vi "Write WebSocket Server Enqueuer.vi"(8 "error in (no error)":errorcluster, 10 "Actor Framework:Message Enqueuer":refnum<class "Message Enqueuer.lvclass">, 11 "WS Test Server in":refnum<class "WS Server Subscriber.lvclass">) -> (0 "error out":errorcluster, 3 "WS Test Server out":refnum<class "WS Server Subscriber.lvclass">)   [LabVIEW 2021, in "Echo Broadcast With Server Manager.lvlib" / "WS Server Subscriber.lvclass"]
uses:
  WS Server Subscriber.lvclass
  <vilib>/ActorFramework/Message Enqueuer/Message Enqueuer.lvclass
  WS Server Subscriber.lvclass/WS Server Subscriber.ctl
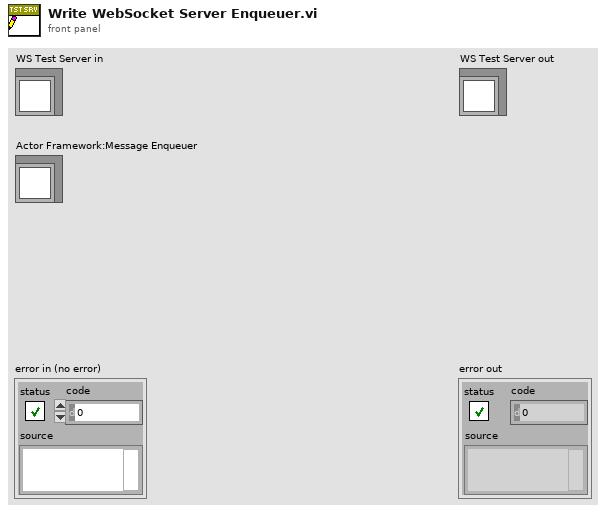
[diagram p1: front panel]
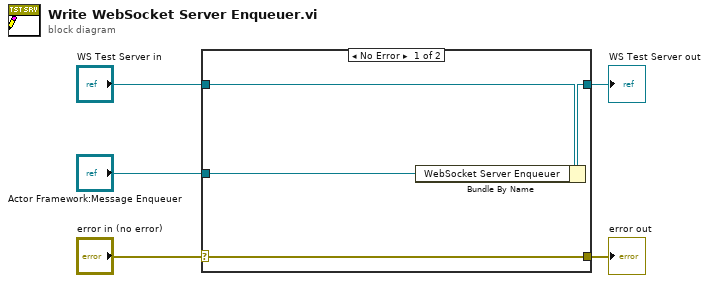
[diagram p0: block diagram]
diagram:
  n1 = case shown="No Error" "error in (no error)" {
    selector: "error in (no error)" -> [w9 w10]
    tunnel: [w9 w10] -> w4
    tunnel: [w7 w11] -> w2
    tunnel: "WS Test Server in" -> [w8 w11]
    tunnel: "Actor Framework:Message Enqueuer" -> [w6 _]
    frame No Error {
      n2 = Bundle By Name(cluster=w8, "WebSocket Server Enqueuer"=w6) -> (w7:refnum<class "WS Server Subscriber.lvclass">)
    }
    frame Error {
    }
  }
  "error out" <- w4
  "WS Test Server out" <- w2
